vi "List.vi"() -> ()   [LabVIEW 2013]
uses:
  <vilib>/Utility/file.llb/Read From Spreadsheet File (string).vi
  <vilib>/Utility/file.llb/Write To Spreadsheet File (string).vi
panel:
  in  "Items":cluster{"Boolean":bool, "String":string}[](array[cluster])
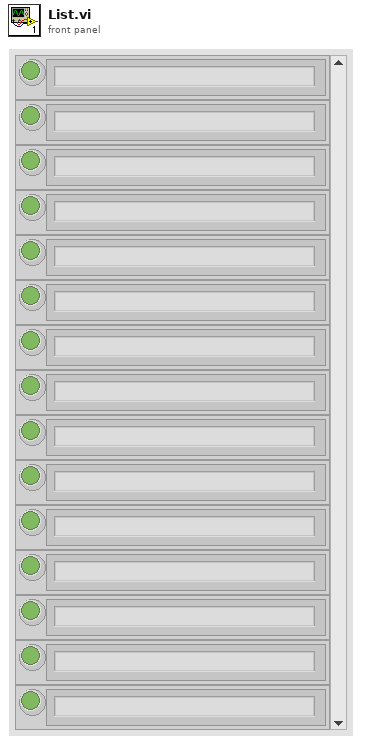
[diagram p1: front panel]
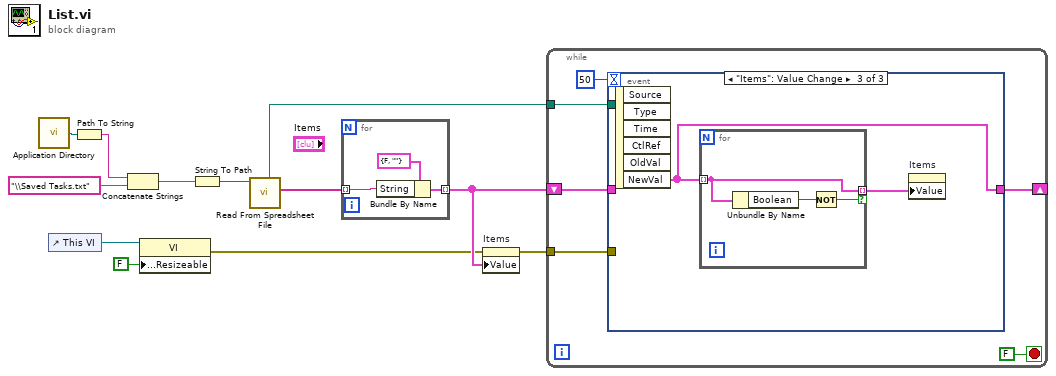
[diagram p0: block diagram]
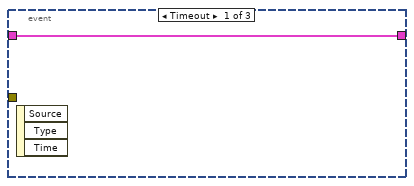
[diagram p2: hidden frame]
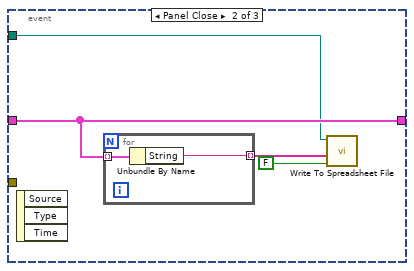
[diagram p3: hidden frame]
diagram:
  n1 = call <vilib>:"Application Directory.vi"() -> ("Application Directory"=w10:path)
  n2 = control-ref of="This VI"() -> (w12:refnum<vi>)
  n3 = Path To String(path=w10) -> (string=w9:string)
  n4 = Concatenate Strings(w9, "\\Saved Tasks.txt" ("string")) -> (w8:string)
  n5 = property class="VI"(reference=w12, "Front Panel.Resizeable"=FALSE ("Front Panel Window:Resizable")) -> (error out=w2:errorcluster)  [unwired: 1 in, 1 out]
  n6 = String To Path(string=w8) -> (path=w6:path)
  n7 = call-poly <vilib>:"Read From Spreadsheet File.vi"("file path (dialog if empty)"=w6) -> ("first row"=w5:string[], "new file path (Not A Path if cancelled)"=w4:path)  [unwired: 6 in, 3 out]
  n8 = for {
    tunnel: w5 -> [w14] mode=indexing
    tunnel: [w15] -> w3 mode=indexing
    n9 = Bundle By Name(cluster=cluster{"Boolean":bool, "String":string} {"Boolean"=FALSE, "String"=""} ("Cluster"), "String"=w14) -> (w15:cluster{"Boolean":bool, "String":string})
  }
  n10 = property on="Items" class="Arr (strict)"(error in=w2, "Value"=w3) -> (error out=w1:errorcluster)  [unwired: 1 in, 1 out]
  n11 = while {
    shift-right: [w19] -> _
    shift-left: w3 -> [w20]
    tunnel: w1 -> [w17]
    tunnel: w4 -> [w16]
    stop <- FALSE stop-if-true
    n12 = event shown="[2] \"Items\": Value Change" {
      selector: _ -> [_ _ _]
      dyn-events: _ -> [_ _ _]
      timeout: 50 -> [_ _ _]
      tunnel: w20 -> [w22 w26 _]
      tunnel: [w22 w26 w30] -> w19
      tunnel: w17 -> [_ _ _]
      tunnel: w16 -> [_ w23 _]
      event Timeout {
        n13 = event-data() -> ()  [unwired: 1 in, 3 out]
      }
      event Panel Close {
        n14 = event-data() -> ()  [unwired: 1 in, 3 out]
        n15 = for {
          tunnel: w26 -> [w28] mode=indexing
          tunnel: [w27] -> w25 mode=indexing
          n16 = Unbundle By Name(w28) -> ("String"=w27:string)
        }
        n17 = call-poly <vilib>:"Write To Spreadsheet File.vi"("append to file? (new file:F)"=FALSE, "1D data"=w25, "file path (dialog if empty)"=w23) -> ()  [unwired: 5 in, 1 out]
      }
      event "Items": Value Change {
        n18 = event-data() -> ("NewVal"=w30:cluster{"Boolean":bool, "String":string}[])  [unwired: 1 in, 5 out]
        n19 = for {
          tunnel: w30 -> [w33] mode=indexing
          tunnel: [w33] -> w29 mode=indexing if=w31
          n20 = Unbundle By Name(w33) -> ("Boolean"=w32:bool)
          n21 = Not(x=w32) -> (.not. x?=w31:bool)
        }
        n22 = property on="Items" class="Arr (strict)"("Value"=w29) -> ()  [unwired: 2 in, 2 out]
      }
    }
  }
